vi "Check Notebook Status Before Quitting App.vi"(8 "Error In":errorcluster, 11 "App name":string) -> (0 "Error Out":errorcluster, 3 "Quit App?":bool)   [LabVIEW 2021, in "Notebook.lvlib"]
uses:
  Notebook.lvlib
  Notebook Parameters List.ctl
  Variant/Variant to Data/Variant to Boolean.vi
  Variant/Variant to Data/Variant to Data.lvlib
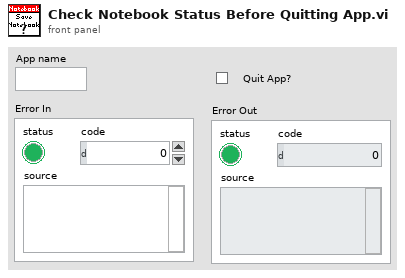
[diagram p1: front panel]
types:
  T1 = typedef "Notebook.lvlib/Notebook Parameters List.ctl" = enum16{"First Opening?", "Saved Notebook?", "Saved Notebook Path", "Beep on Error?"}
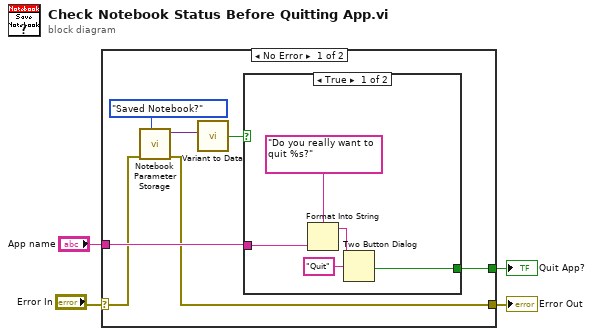
[diagram p0: block diagram]
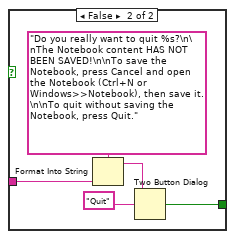
[diagram p2: hidden frame]
diagram:
  n1 = case shown="No Error" "Error In" {
    selector: "Error In" -> [w6 w22]
    tunnel: "App name" -> [w7 _]
    tunnel: [w11 _] -> w3
    tunnel: [w5 w22] -> w1
    frame No Error {
      n2 = call "Notebook Parameter Storage.vi"("Notebook Parameter List"=Notebook_Parameters_List."Saved Notebook?", "Error In"=w6) -> ("Error Out"=w5:errorcluster, "Data out"=w10:variant)  [unwired: 8 in]
      n3 = call-poly "Variant to Data.vi"("Variant"=w10) -> ("Value"=w8:bool)  [unwired: 8 in]
      n4 = case shown="True" w8 {
        tunnel: [w14 w21] -> w11
        tunnel: w7 -> [w12 w17]
        frame True {
          n5 = Format Into String(format string="Do you really want to quit %s?" ("message"), w12) -> (resulting string=w13:string)  [unwired: 2 in, 1 out]
          n6 = Two Button Dialog(message=w13, 2:"Quit" ("T button name (\"OK\")")) -> (T button?=w14:bool)  [unwired: 1 in]
        }
        frame False {
          n7 = Format Into String(format string="Do you really want to quit %s?\n\nThe Notebook content HAS NOT BEEN SAVED!\n\nTo save the Notebook, press Cancel and open the Notebook (Ctrl+N or Windows>>Notebook), then save it.\n\nTo quit without saving the Notebook, press Quit." ("message"), w17) -> (resulting string=w18:string)  [unwired: 2 in, 1 out]
          n8 = Two Button Dialog(message=w18, 2:"Quit" ("T button name (\"OK\")")) -> (T button?=w21:bool)  [unwired: 1 in]
        }
      }
    }
    frame Error {
    }
  }
  "Quit App?" <- w3
  "Error Out" <- w1
